vi "Prompting.vi"(5 "New Integration Time":i32, 7 "Command":T1, 8 "error in (no error)":errorcluster, 9 "Type":string, 10 "Wafer ID":string, 11 "EpiWrapper in":refnum<class "EpiWrapper.lvclass">) -> (0 "error out":errorcluster, 3 "EpiWrapper out":refnum<class "EpiWrapper.lvclass">)   [LabVIEW 2012, in "EpiWrapper.lvclass"]
uses:
  EpiWrapper.lvclass
  Controls/Command_Enum.ctl
  EpiWrapper.lvclass/EpiWrapper.ctl
  LotData.lvclass
  Controls/TestArea.ctl
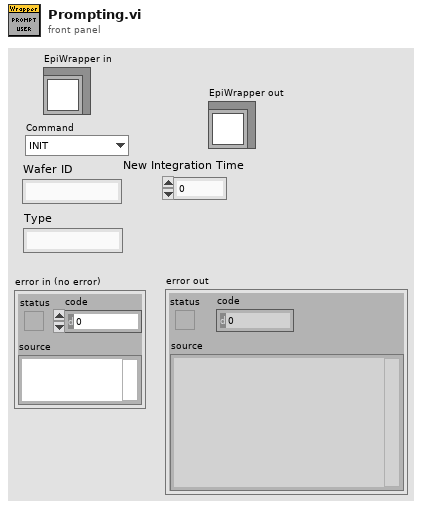
[diagram p1: front panel]
types:
  T1 = typedef "Command_Enum.ctl" = enum16{"INIT", "LOAD", "MEASURE", "NEW", "SAVE", "SWAP_MODE", "UPDATE_ACQ", "EXIT", "CANCEL"}
  T2 = enum8{"Enabled", "Disabled", "Disabled and Grayed Out"}
  T3 = typedef "TestArea.ctl" = string
  T4 = typedef "MeasureControl.ctl" = cluster{"Pass":bool, "Fail":bool, "Measure":bool, "Area":T3, "TestData":T5, "Graph":cluster{"Y":dbl[], "Y":dbl[]}[]}
  T5 = typedef "TestData.ctl" = cluster{"20mA Data":cluster{"Area":string, "Current,mA":dbl, "Power":dbl, "WL":dbl, "Voltage":dbl, "Knee Current":dbl, "Reverse":dbl}, "50mA Data":cluster{"Area":string, "Current,mA":dbl, "Power":dbl, "WL":dbl, "Voltage":dbl}}
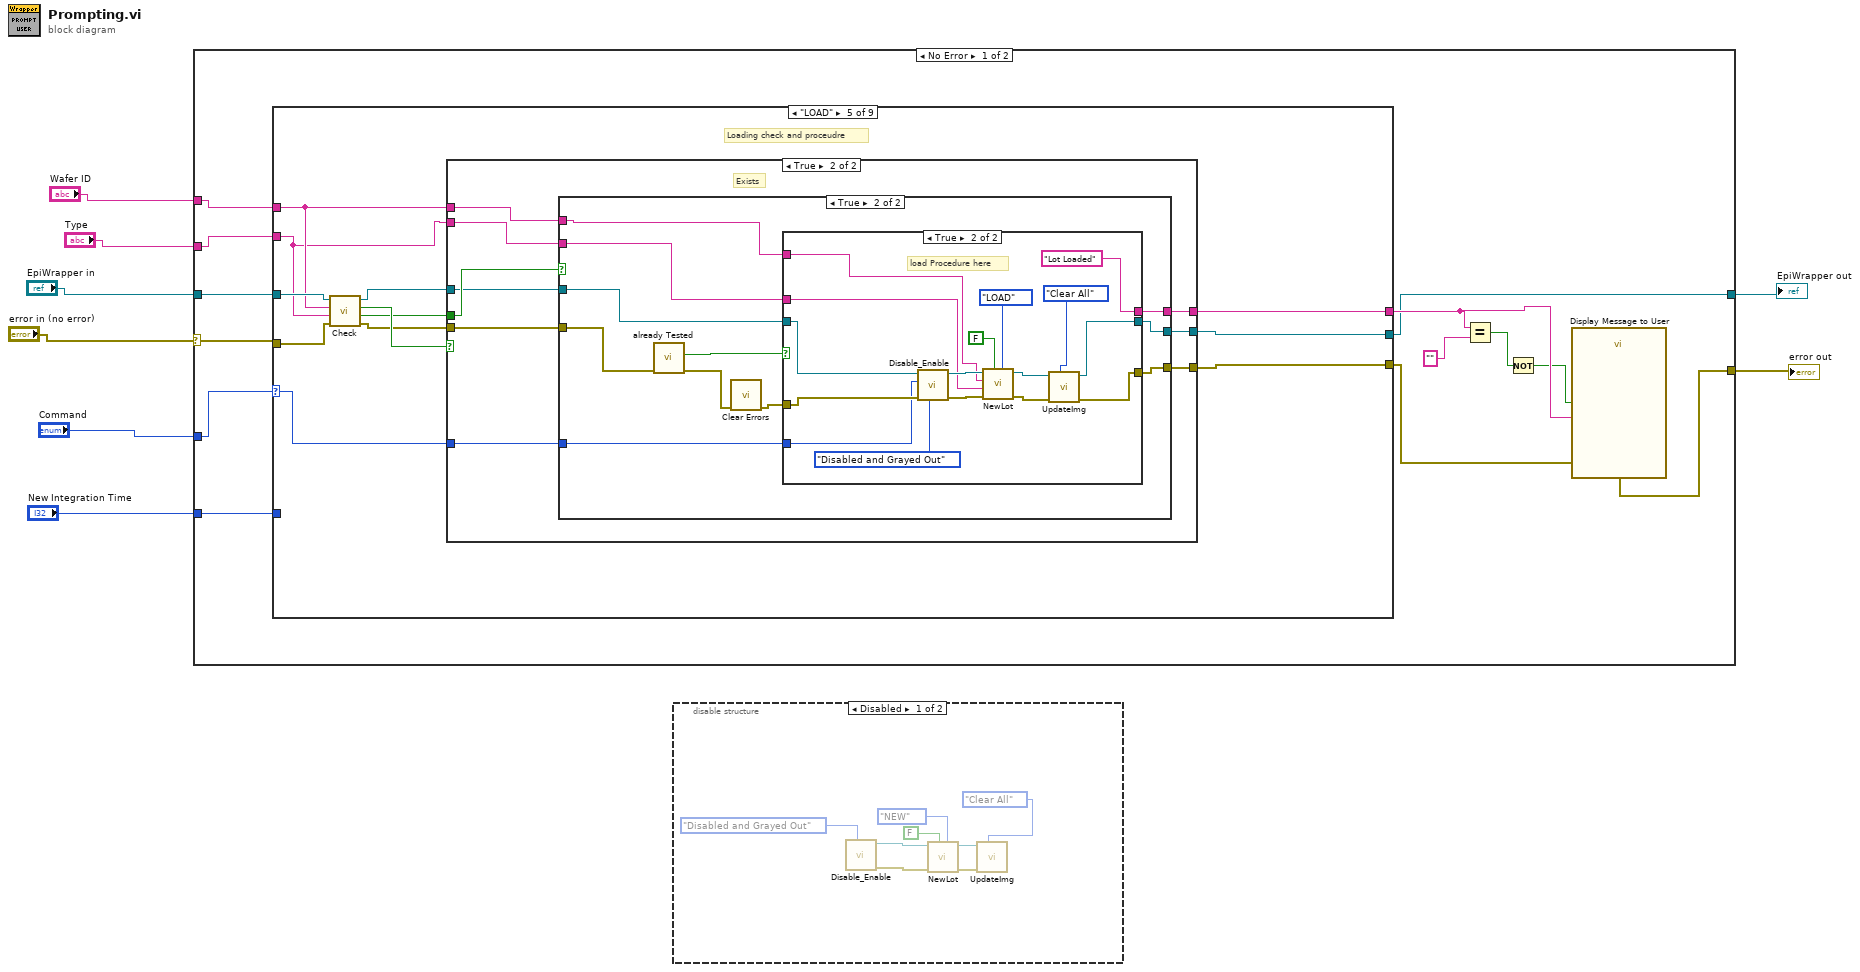
[diagram p0: block diagram]
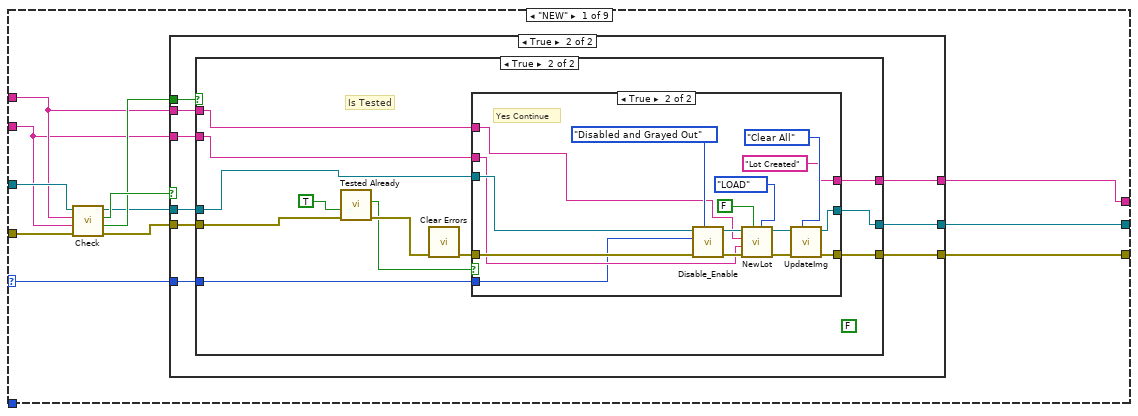
[diagram p3: hidden frame]
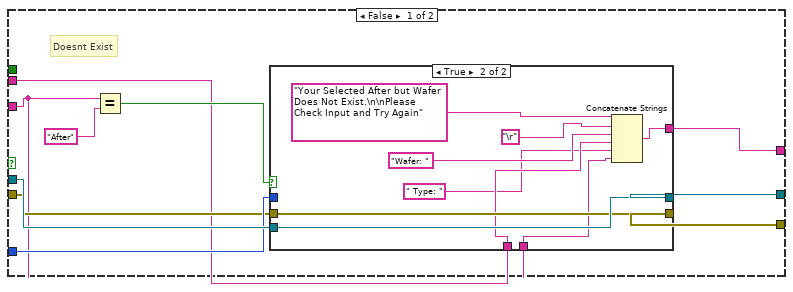
[diagram p4: hidden frame]
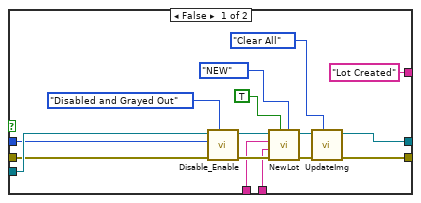
[diagram p5: hidden frame]
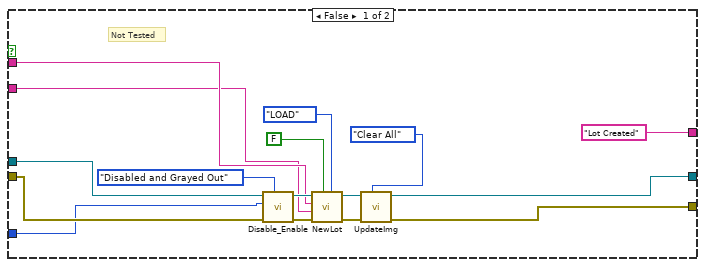
[diagram p6: hidden frame]
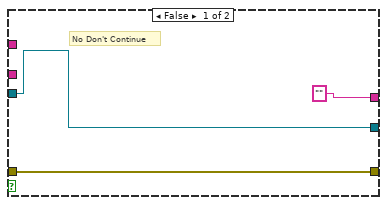
[diagram p7: hidden frame]
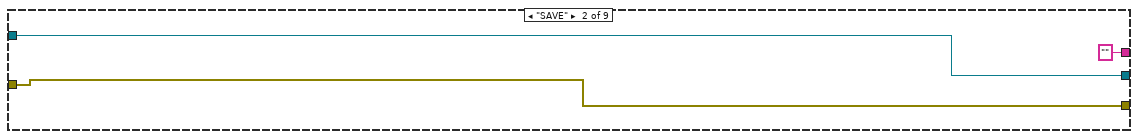
[diagram p8: hidden frame]
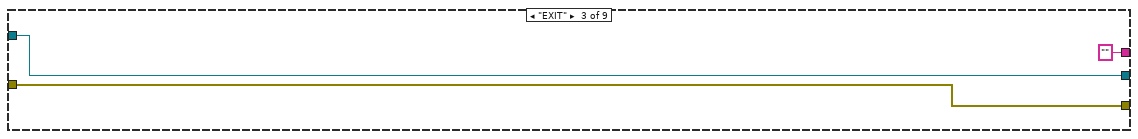
[diagram p9: hidden frame]
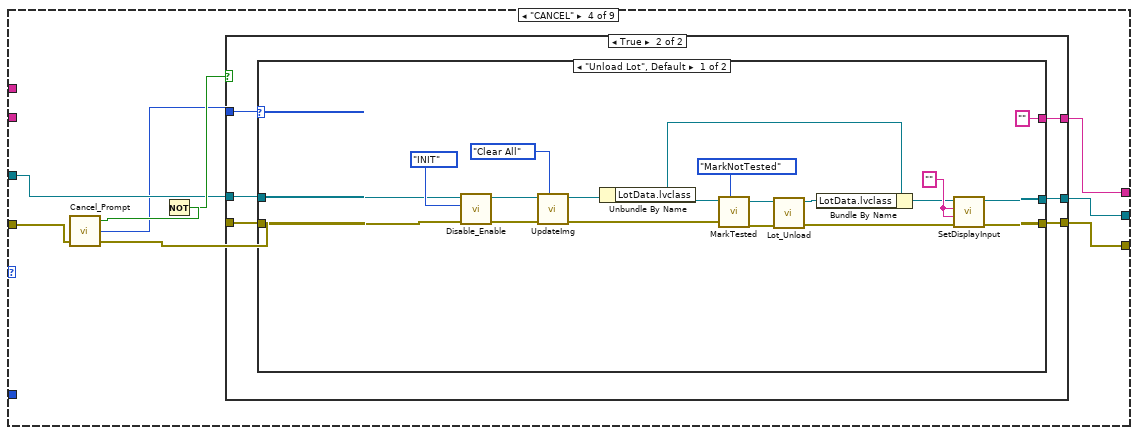
[diagram p10: hidden frame]
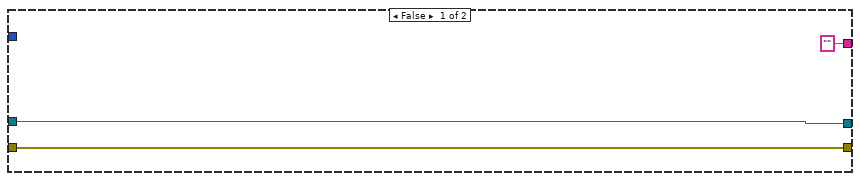
[diagram p11: hidden frame]
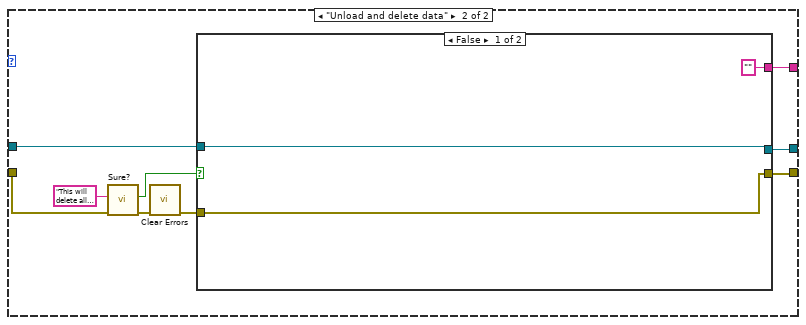
[diagram p12: hidden frame]
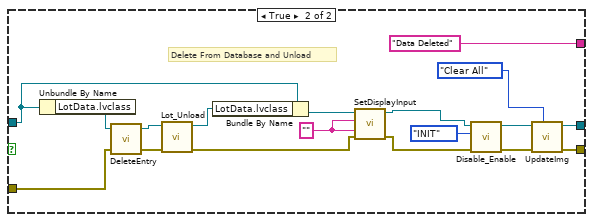
[diagram p13: hidden frame]
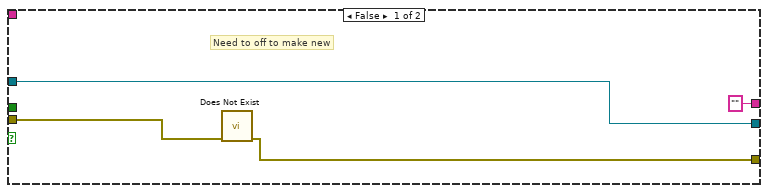
[diagram p14: hidden frame]
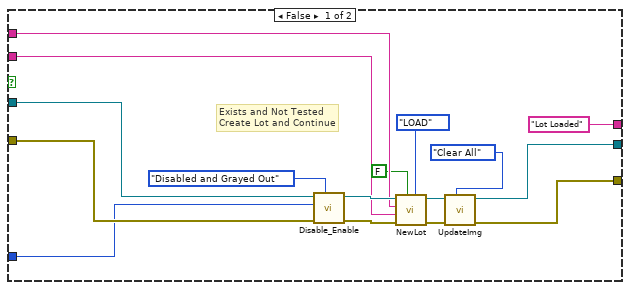
[diagram p15: hidden frame]
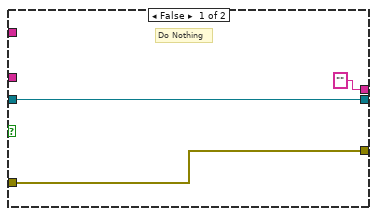
[diagram p16: hidden frame]
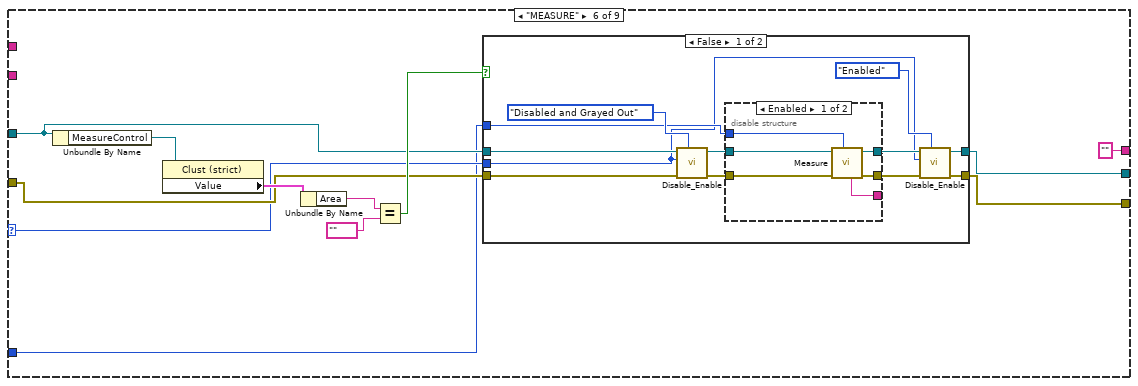
[diagram p17: hidden frame]
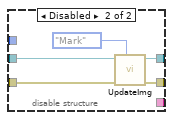
[diagram p18: hidden frame]
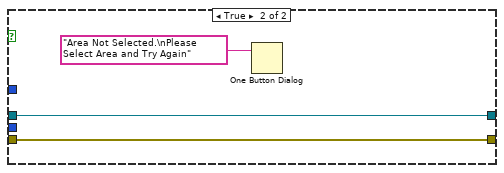
[diagram p19: hidden frame]
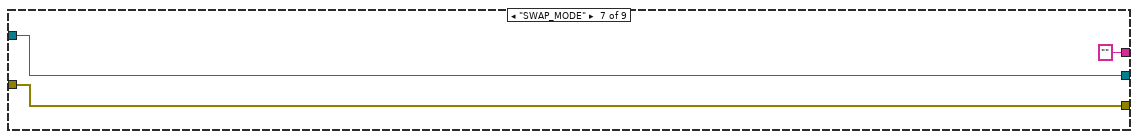
[diagram p20: hidden frame]
diagram:
  n1 = case shown="No Error" "error in (no error)" {
    selector: "error in (no error)" -> [w17 w317]
    tunnel: [w11 w317] -> w7
    tunnel: [w10 w316] -> w5
    tunnel: "EpiWrapper in" -> [w20 w316]
    tunnel: "Wafer ID" -> [w19 _]
    tunnel: "Type" -> [w18 _]
    tunnel: "Command" -> [w21 _]
    tunnel: "New Integration Time" -> [w9 _]
    frame No Error {
      n2 = case shown="\"LOAD\"" w21 {
        selector: w21 -> [w26 _ _ _ w199 w270 _ _ _]
        tunnel: [w33 w126 w129 w135 w200 w272 w308 w311 w314] -> w12
        tunnel: w20 -> [w32 w127 w130 w136 w209 w274 w309 w312 w315]
        tunnel: w19 -> [w25 _ _ _ w205 _ _ _ _]
        tunnel: w18 -> [w24 _ _ _ w204 _ _ _ _]
        tunnel: w17 -> [w31 w126 w129 w139 w208 w273 w308 w311 w314]
        tunnel: [w23 w127 w130 w133 w201 w271 w309 w312 w315] -> w10
        tunnel: [w22 "" "" w131 w198 "" "" "" ""] -> w15
        tunnel: w9 -> [_ _ _ _ _ w269 _ _ _]
        frame "NEW" {
          n3 = call-dynamic "Check.vi"("error in (no error)"=w31, "Type"=w24, "Wafer ID"=w25, "EpiWrapper in"=w32) -> ("error out"=w28:errorcluster, "Tested?"=w29:bool, "Exists?"=w30:bool, "EpiWrapper out"=w27:refnum<class "EpiWrapper.lvclass">)  [unwired: 4 in]
          n4 = case shown="True" w30 {
            tunnel: [w42 w77] -> w33
            tunnel: w29 -> [_ w76]
            tunnel: w28 -> [w37 w75]
            tunnel: w27 -> [w39 w74]
            tunnel: w26 -> [w38 w73]
            tunnel: w25 -> [w35 w72]
            tunnel: w24 -> [w34 w71]
            tunnel: [w43 w70] -> w23
            tunnel: [w36 w69] -> w22
            frame False {
              # "Doesnt Exist"
              n5 = Equal?(x=w34, y="After" ("Type")) -> (x = y?=w40:bool)
              n6 = case shown="True" w40 {
                tunnel: [w51 w68] -> w43
                tunnel: [w50 w67] -> w42
                tunnel: w39 -> [w49 w68]
                tunnel: w38 -> [w48 _]
                tunnel: w37 -> [w47 w67]
                tunnel: ["Lot Created" w60] -> w36
                tunnel: w35 -> [w45 w63]
                tunnel: w34 -> [w44 w61]
                frame False {
                  n7 = call-dynamic "Disable_Enable.vi"("Disabled"=T2."Disabled and Grayed Out", "error in (no error)"=w47, "Command"=w48, "EpiWrapper in"=w49) -> ("error out"=w56:errorcluster, "EpiWrapper out"=w58:refnum<class "EpiWrapper.lvclass">)  [unwired: 6 in]
                  n8 = call-dynamic "NewLot.vi"("Enum"=enum16{"LOAD", "NEW"}."NEW", "Create Entry?"=TRUE, "error in (no error)"=w56, "Test"=w44, "Wafer ID"=w45, "FrontPanelData in"=w58) -> ("error out"=w57:errorcluster, "FrontPanelData out"=w59:refnum<class "EpiWrapper.lvclass">)  [unwired: 3 in, 1 out]
                  n9 = call-dynamic "UpdateImg.vi"("Enum"=enum16{"Mark", "Clear All"}."Clear All", "error in (no error)"=w57, "EpiWrapper in"=w59) -> ("error out"=w50:errorcluster, "EpiWrapper out"=w51:refnum<class "EpiWrapper.lvclass">)  [unwired: 7 in]
                }
                frame True {
                  n10 = Concatenate Strings("Your Selected After but Wafer Does Not Exist.\n\nPlease Check Input and Try Again", "\r", "Wafer: " ("string"), w63, " Type: " ("string"), w61) -> (w60:string)
                }
              }
            }
            frame True {
              n11 = case shown="True" w76 {
                tunnel: w75 -> [w92 w103]
                tunnel: [w93 w100] -> w77
                tunnel: w74 -> [w87 w99]
                tunnel: w73 -> [w86 w95]
                tunnel: w72 -> [w84 w97]
                tunnel: w71 -> [w83 w96]
                tunnel: [w81 w98] -> w70
                tunnel: ["Lot Created" w94] -> w69
                frame False {
                  # "Not Tested"
                  n12 = call-dynamic "Disable_Enable.vi"("Disabled"=T2."Disabled and Grayed Out", "error in (no error)"=w92, "Command"=w86, "EpiWrapper in"=w87) -> ("error out"=w89:errorcluster, "EpiWrapper out"=w85:refnum<class "EpiWrapper.lvclass">)  [unwired: 6 in]
                  n13 = call-dynamic "NewLot.vi"("Enum"=enum16{"LOAD", "NEW"}."LOAD", "Create Entry?"=FALSE, "error in (no error)"=w89, "Test"=w83, "Wafer ID"=w84, "FrontPanelData in"=w85) -> ("error out"=w88:errorcluster, "FrontPanelData out"=w82:refnum<class "EpiWrapper.lvclass">)  [unwired: 3 in, 1 out]
                  n14 = call-dynamic "UpdateImg.vi"("Enum"=enum16{"Mark", "Clear All"}."Clear All", "error in (no error)"=w88, "EpiWrapper in"=w82) -> ("error out"=w93:errorcluster, "EpiWrapper out"=w81:refnum<class "EpiWrapper.lvclass">)  [unwired: 7 in]
                }
                frame True {
                  (unwired) FALSE ("T button?")
                  # "Is Tested"
                  n15 = call "Tested Already"("error in (no error)"=w103, "Enable"=TRUE) -> ("error out"=w105:errorcluster, "Continue"=w104:bool)  [unwired: 8 in]
                  n16 = call <vilib>:"Clear Errors.vi"("error in (no error)"=w105) -> ("error out"=w101:errorcluster)  [unwired: 6 in]
                  n17 = case shown="True" w104 {
                    tunnel: w101 -> [w108 w122]
                    tunnel: [w108 w119] -> w100
                    tunnel: w99 -> [w107 w115]
                    tunnel: [w107 w114] -> w98
                    tunnel: w97 -> [_ w112]
                    tunnel: w96 -> [_ w111]
                    tunnel: w95 -> [_ w110]
                    tunnel: ["" "Lot Created"] -> w94
                    frame False {
                      # "No Don't Continue"
                    }
                    frame True {
                      # "Yes Continue"
                      n18 = call-dynamic "Disable_Enable.vi"("Disabled"=T2."Disabled and Grayed Out", "error in (no error)"=w122, "Command"=w110, "EpiWrapper in"=w115) -> ("error out"=w121:errorcluster, "EpiWrapper out"=w116:refnum<class "EpiWrapper.lvclass">)  [unwired: 6 in]
                      n19 = call-dynamic "NewLot.vi"("Enum"=enum16{"LOAD", "NEW"}."LOAD", "Create Entry?"=FALSE, "error in (no error)"=w121, "Test"=w111, "Wafer ID"=w112, "FrontPanelData in"=w116) -> ("error out"=w120:errorcluster, "FrontPanelData out"=w117:refnum<class "EpiWrapper.lvclass">)  [unwired: 3 in, 1 out]
                      n20 = call-dynamic "UpdateImg.vi"("Enum"=enum16{"Mark", "Clear All"}."Clear All", "error in (no error)"=w120, "EpiWrapper in"=w117) -> ("error out"=w119:errorcluster, "EpiWrapper out"=w114:refnum<class "EpiWrapper.lvclass">)  [unwired: 7 in]
                    }
                  }
                }
              }
            }
          }
        }
        frame "SAVE" {
        }
        frame "EXIT" {
        }
        frame "CANCEL" {
          n21 = call "Cancel_Prompt.vi"("error in (no error)"=w139) -> ("error out"=w134:errorcluster, "Enum 2"=w132:enum16{"Unload Lot", "Unload and delete data"}, "Cancelled?"=w138:bool)  [unwired: 2 in]
          n22 = Not(x=w138) -> (.not. x?=w137:bool)
          n23 = case shown="True" w137 {
            tunnel: w132 -> [_ w148]
            tunnel: w136 -> [w142 w147]
            tunnel: [w141 w145] -> w135
            tunnel: w134 -> [w141 w146]
            tunnel: [w142 w144] -> w133
            tunnel: ["" w143] -> w131
            frame False {
            }
            frame True {
              n24 = case shown="\"Unload Lot\", Default" w148 {
                tunnel: w147 -> [w164 w176]
                tunnel: w146 -> [w163 w171]
                tunnel: [w152 w175] -> w145
                tunnel: [w153 w174] -> w144
                tunnel: ["" w168] -> w143
                frame "Unload Lot", Default {
                  w154 = "" ("Wafer ID")
                  n25 = call-dynamic "Disable_Enable.vi"("error in (no error)"=w163, "Command"=Command_Enum."INIT", "EpiWrapper in"=w164) -> ("error out"=w165:errorcluster, "EpiWrapper out"=w166:refnum<class "EpiWrapper.lvclass">)  [unwired: 7 in]
                  n26 = call-dynamic "UpdateImg.vi"("Enum"=enum16{"Mark", "Clear All"}."Clear All", "error in (no error)"=w165, "EpiWrapper in"=w166) -> ("error out"=w155:errorcluster, "EpiWrapper out"=w156:refnum<class "EpiWrapper.lvclass">)  [unwired: 7 in]
                  n27 = Unbundle By Name(w156) -> ("LotData.lvclass"=w157:refnum<class "LotData.lvclass">)
                  n28 = call-dynamic "MarkTested.vi"("Enum"=enum16{"MarkTested", "MarkNotTested"}."MarkNotTested", "error in (no error)"=w155, "LotData in"=w157) -> ("error out"=w159:errorcluster, "LotData out"=w160:refnum<class "LotData.lvclass">)  [unwired: 6 in, 1 out]
                  n29 = call-dynamic "Lot_Unload.vi"("error in (no error)"=w159, "LotData in"=w160) -> ("error out"=w150:errorcluster, "LotData out"=w161:refnum<class "LotData.lvclass">)  [unwired: 8 in]
                  n30 = Bundle By Name(cluster=w156, "LotData.lvclass"=w161) -> (w151:refnum<class "EpiWrapper.lvclass">)
                  n31 = call-dynamic "SetDisplayInput.vi"("error in (no error)"=w150, "Test"=w154, "Wafer ID"=w154, "EpiWrapper in"=w151) -> ("error out"=w152:errorcluster, "EpiWrapper out"=w153:refnum<class "EpiWrapper.lvclass">)  [unwired: 6 in]
                }
                frame "Unload and delete data" {
                  n32 = call "Sure?"("error in (no error)"=w171, "Message"="This will delete all data associated with this wafer.\n\nAre you absolutly sure you want to continue?") -> ("error out"=w172:errorcluster, "YES,DELETE DATA"=w170:bool)  [unwired: 8 in]
                  n33 = call <vilib>:"Clear Errors.vi"("error in (no error)"=w172) -> ("error out"=w169:errorcluster)  [unwired: 6 in]
                  n34 = case shown="False" w170 {
                    tunnel: w176 -> [w179 w190]
                    tunnel: [w178 w188] -> w175
                    tunnel: [w179 w187] -> w174
                    tunnel: w169 -> [w178 w181]
                    tunnel: ["" "Data Deleted"] -> w168
                    frame False {
                    }
                    frame True {
                      w185 = "" ("Wafer ID")
                      # "Delete From Database and Unload"
                      n35 = Unbundle By Name(w190) -> ("LotData.lvclass"=w193:refnum<class "LotData.lvclass">)
                      n36 = call-dynamic "DeleteEntry.vi"("error in (no error)"=w181, "LotData in"=w193) -> ("error out"=w191:errorcluster, "LotData out"=w192:refnum<class "LotData.lvclass">)  [unwired: 1 in, 1 out]
                      n37 = call-dynamic "Lot_Unload.vi"("error in (no error)"=w191, "LotData in"=w192) -> ("error out"=w184:errorcluster, "LotData out"=w189:refnum<class "LotData.lvclass">)  [unwired: 8 in]
                      n38 = Bundle By Name(cluster=w190, "LotData.lvclass"=w189) -> (w186:refnum<class "EpiWrapper.lvclass">)
                      n39 = call-dynamic "SetDisplayInput.vi"("error in (no error)"=w184, "Test"=w185, "Wafer ID"=w185, "EpiWrapper in"=w186) -> ("error out"=w183:errorcluster, "EpiWrapper out"=w182:refnum<class "EpiWrapper.lvclass">)  [unwired: 6 in]
                      n40 = call-dynamic "Disable_Enable.vi"("error in (no error)"=w183, "Command"=Command_Enum."INIT", "EpiWrapper in"=w182) -> ("error out"=w195:errorcluster, "EpiWrapper out"=w196:refnum<class "EpiWrapper.lvclass">)  [unwired: 7 in]
                      n41 = call-dynamic "UpdateImg.vi"("Enum"=enum16{"Mark", "Clear All"}."Clear All", "error in (no error)"=w195, "EpiWrapper in"=w196) -> ("error out"=w188:errorcluster, "EpiWrapper out"=w187:refnum<class "EpiWrapper.lvclass">)  [unwired: 7 in]
                    }
                  }
                }
              }
            }
          }
        }
        frame "LOAD" {
          # "Loading check and proceudre"
          n42 = call-dynamic "Check.vi"("error in (no error)"=w208, "Type"=w204, "Wafer ID"=w205, "EpiWrapper in"=w209) -> ("error out"=w202:errorcluster, "Tested?"=w206:bool, "Exists?"=w207:bool, "EpiWrapper out"=w203:refnum<class "EpiWrapper.lvclass">)  [unwired: 4 in]
          n43 = case shown="True" w207 {
            tunnel: w206 -> [_ w222]
            tunnel: w205 -> [_ w221]
            tunnel: w204 -> [_ w220]
            tunnel: w203 -> [w211 w219]
            tunnel: w202 -> [w213 w218]
            tunnel: [w211 w217] -> w201
            tunnel: [w212 w216] -> w200
            tunnel: w199 -> [_ w215]
            tunnel: ["" w214] -> w198
            frame False {
              # "Need to off to make new"
              n44 = call "Does Not Exist"("error in (no error)"=w213) -> ("error out"=w212:errorcluster)  [unwired: 9 in, 1 out]
            }
            frame True {
              # "Exists"
              n45 = case shown="True" w222 {
                tunnel: w221 -> [w232 w240]
                tunnel: w220 -> [w231 w239]
                tunnel: w219 -> [w230 w244]
                tunnel: w218 -> [w229 w243]
                tunnel: [w228 w245] -> w217
                tunnel: [w227 w247] -> w216
                tunnel: w215 -> [w224 w242]
                tunnel: ["Lot Loaded" w241] -> w214
                frame False {
                  # "Exists and Not Tested\nCreate Lot and Continue"
                  n46 = call-dynamic "Disable_Enable.vi"("Disabled"=T2."Disabled and Grayed Out", "error in (no error)"=w229, "Command"=w224, "EpiWrapper in"=w230) -> ("error out"=w236:errorcluster, "EpiWrapper out"=w234:refnum<class "EpiWrapper.lvclass">)  [unwired: 6 in]
                  n47 = call-dynamic "NewLot.vi"("Enum"=enum16{"LOAD", "NEW"}."LOAD", "Create Entry?"=FALSE, "error in (no error)"=w236, "Test"=w231, "Wafer ID"=w232, "FrontPanelData in"=w234) -> ("error out"=w235:errorcluster, "FrontPanelData out"=w233:refnum<class "EpiWrapper.lvclass">)  [unwired: 3 in, 1 out]
                  n48 = call-dynamic "UpdateImg.vi"("Enum"=enum16{"Mark", "Clear All"}."Clear All", "error in (no error)"=w235, "EpiWrapper in"=w233) -> ("error out"=w227:errorcluster, "EpiWrapper out"=w228:refnum<class "EpiWrapper.lvclass">)  [unwired: 7 in]
                }
                frame True {
                  n49 = call "already Tested"("error in (no error)"=w243) -> ("error out"=w248:errorcluster, "Continue"=w249:bool)  [unwired: 9 in]
                  n50 = call <vilib>:"Clear Errors.vi"("error in (no error)"=w248) -> ("error out"=w246:errorcluster)  [unwired: 6 in]
                  n51 = case shown="True" w249 {
                    tunnel: [w252 w261] -> w247
                    tunnel: w246 -> [w252 w259]
                    tunnel: [w251 w262] -> w245
                    tunnel: w244 -> [w251 w260]
                    tunnel: w240 -> [_ w258]
                    tunnel: w239 -> [_ w257]
                    tunnel: w242 -> [_ w254]
                    tunnel: ["" "Lot Loaded"] -> w241
                    frame False {
                      # "Do Nothing"
                    }
                    frame True {
                      # "load Procedure here"
                      n52 = call-dynamic "Disable_Enable.vi"("Disabled"=T2."Disabled and Grayed Out", "error in (no error)"=w259, "Command"=w254, "EpiWrapper in"=w260) -> ("error out"=w265:errorcluster, "EpiWrapper out"=w267:refnum<class "EpiWrapper.lvclass">)  [unwired: 6 in]
                      n53 = call-dynamic "NewLot.vi"("Enum"=enum16{"LOAD", "NEW"}."LOAD", "Create Entry?"=FALSE, "error in (no error)"=w265, "Test"=w257, "Wafer ID"=w258, "FrontPanelData in"=w267) -> ("error out"=w266:errorcluster, "FrontPanelData out"=w268:refnum<class "EpiWrapper.lvclass">)  [unwired: 3 in, 1 out]
                      n54 = call-dynamic "UpdateImg.vi"("Enum"=enum16{"Mark", "Clear All"}."Clear All", "error in (no error)"=w266, "EpiWrapper in"=w268) -> ("error out"=w261:errorcluster, "EpiWrapper out"=w262:refnum<class "EpiWrapper.lvclass">)  [unwired: 7 in]
                    }
                  }
                }
              }
            }
          }
        }
        frame "MEASURE" {
          n55 = Unbundle By Name(w274) -> ("MeasureControl"=w279:refnum<vi>)
          n56 = property class="Clust (strict)"(reference=w279) -> ("Value"=w278:T4)  [unwired: 1 in, 2 out]
          n57 = Unbundle By Name(w278) -> ("Area"=w277:T3)
          n58 = Equal?(x=w277, y=T3 "") -> (x = y?=w275:bool)
          n59 = case shown="False" w275 {
            tunnel: w274 -> [w286 w305]
            tunnel: w273 -> [w285 w304]
            tunnel: [w284 w304] -> w272
            tunnel: [w283 w305] -> w271
            tunnel: w270 -> [w281 _]
            tunnel: w269 -> [w282 _]
            frame False {
              n60 = call-dynamic "Disable_Enable.vi"("Disabled"=T2."Disabled and Grayed Out", "error in (no error)"=w285, "Command"=w281, "EpiWrapper in"=w286) -> ("error out"=w289:errorcluster, "EpiWrapper out"=w290:refnum<class "EpiWrapper.lvclass">)  [unwired: 6 in]
              n61 = disable-structure shown="Enabled" {
                disable-tunnel: w290 -> [w298 w303]
                disable-tunnel: w289 -> [w297 w302]
                disable-tunnel: [w296 _] -> _
                disable-tunnel: [w295 w301] -> w288
                disable-tunnel: [w294 w300] -> w287
                disable-tunnel: w282 -> [w293 _]
                frame Enabled {
                  n62 = call-dynamic "Measure.vi"("New Integration Time"=w293, "error in (no error)"=w297, "EpiWrapper in"=w298) -> ("error out"=w295:errorcluster, "EpiWrapper out"=w294:refnum<class "EpiWrapper.lvclass">, "ExcelOut"=w296:string)  [unwired: 4 in, 2 out]
                }
                frame Disabled {
                  n63 = call-dynamic "UpdateImg.vi"("Enum"=enum16{"Mark", "Clear All"}."Mark", "error in (no error)"=w302, "EpiWrapper in"=w303) -> ("error out"=w301:errorcluster, "EpiWrapper out"=w300:refnum<class "EpiWrapper.lvclass">)  [unwired: 7 in]
                }
              }
              n64 = call-dynamic "Disable_Enable.vi"("Disabled"=T2."Enabled", "error in (no error)"=w288, "Command"=w281, "EpiWrapper in"=w287) -> ("error out"=w284:errorcluster, "EpiWrapper out"=w283:refnum<class "EpiWrapper.lvclass">)  [unwired: 6 in]
            }
            frame True {
              n65 = One Button Dialog(message="Area Not Selected.\nPlease Select Area and Try Again") -> ()  [unwired: 1 in, 1 out]
            }
          }
        }
        frame "SWAP_MODE" {
        }
        frame "UPDATE_ACQ" {
        }
        frame "INIT" {
        }
      }
      n66 = Equal?(x=w15, y="") -> (x = y?=w14:bool)
      n67 = Not(x=w14) -> (.not. x?=w13:bool)
      n68 = call "Display Message to User"("error in (no error)"=w12, "Enable"=w13, "Message"=w15) -> ("error out"=w11:errorcluster)  [unwired: 7 in, 1 out]
    }
    frame Error {
    }
  }
  "error out" <- w7
  "EpiWrapper out" <- w5
  n69 = disable-structure shown="Disabled" {
    frame Disabled {
      n70 = call-dynamic "Disable_Enable.vi"("Disabled"=T2."Disabled and Grayed Out") -> ("error out"=w322:errorcluster, "EpiWrapper out"=w324:refnum<class "EpiWrapper.lvclass">)  [unwired: 9 in]
      n71 = call-dynamic "NewLot.vi"("Enum"=enum16{"LOAD", "NEW"}."NEW", "Create Entry?"=FALSE, "error in (no error)"=w322, "FrontPanelData in"=w324) -> ("error out"=w323:errorcluster, "FrontPanelData out"=w325:refnum<class "EpiWrapper.lvclass">)  [unwired: 5 in, 1 out]
      n72 = call-dynamic "UpdateImg.vi"("Enum"=enum16{"Mark", "Clear All"}."Clear All", "error in (no error)"=w323, "EpiWrapper in"=w325) -> ()  [unwired: 7 in, 2 out]
    }
    frame Enabled {
    }
  }
